vi "GetFrame.vi"(8 "error in (no error)":errorcluster, 11 "ZWO_ASI in":refnum<class "ZWO_ASI.lvclass">) -> (0 "error out":errorcluster, 3 "ZWO_ASI out":refnum<class "ZWO_ASI.lvclass">)   [LabVIEW 2023, in "ZWO_ASI.lvlib" / "ZWO_ASI.lvclass"]
uses:
  ZWO_ASI.lvclass
  Labview_ASI_demo_64bit_221128/user.lib/ASICamera2_no_err/ASICamera2_no_err.lvlib
  <vilib>/ActorFramework/Actor/Actor.lvclass
  ZWO_ASI Messages/GetFrame Msg/GetFrame Msg.lvclass
  C:/Program Files/National Instruments/LabVIEW 2023/vi.lib/ActorFramework/Actor/Actor.lvclass
  C:/Users/quantum/Documents/LVDAQ/ConcreteClasses/ConcreteInstrumentClasses/CameraClasses/ZWO_ASI_LV/ZWO_ASI/ZWO_ASI.lvclass
  C:/Users/quantum/Documents/LVDAQ/Interfaces/AbstractInstrumentClasses/Cameras_LV/CameraInterface/CameraInterface.lvclass
  C:/Users/quantum/Documents/LVDAQ/Interfaces/InitDeinitInterface/InitDeinit/InitDeinit.lvclass
  ZWO_ASI Messages/StopCapture Msg/StopCapture Msg.lvclass
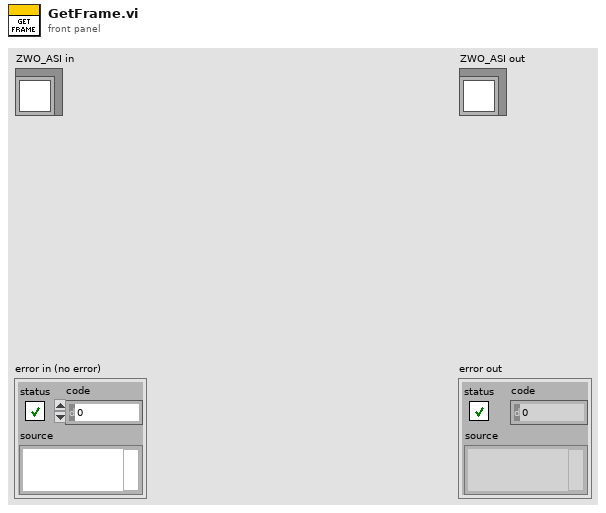
[diagram p1: front panel]
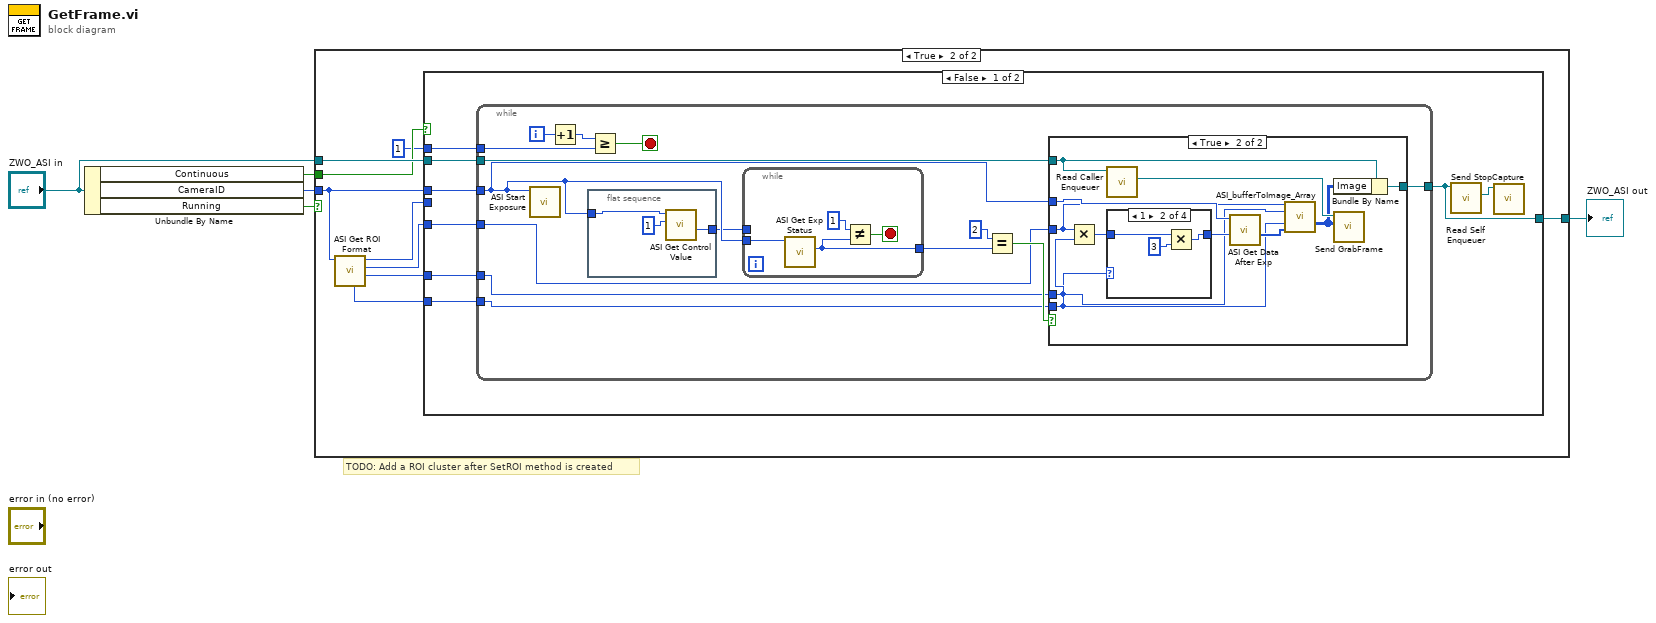
[diagram p0: block diagram]
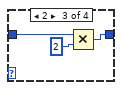
[diagram p5: hidden frame]
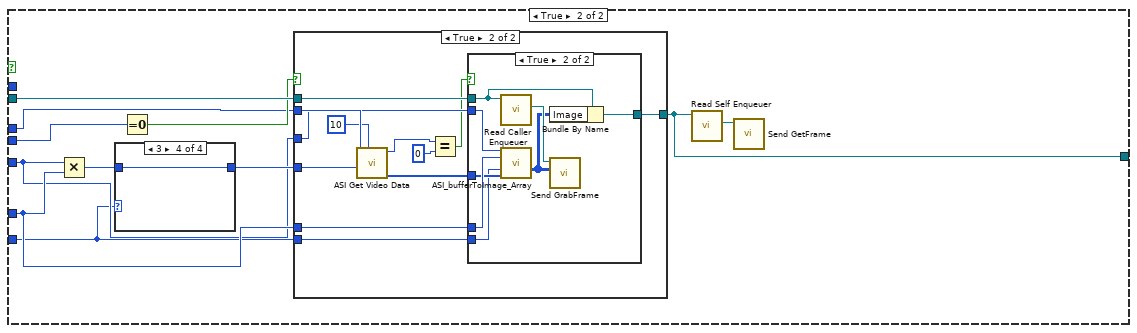
[diagram p7: hidden frame]
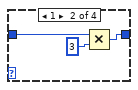
[diagram p11: hidden frame]
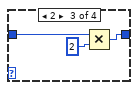
[diagram p12: hidden frame]
diagram:
  # "TODO: Add a ROI cluster after SetROI method is created"
  n1 = Unbundle By Name("ZWO_ASI in") -> ("Continuous"=w4:bool, "CameraID"=w3:i32, "Running"=w2:bool)
  n2 = case shown="True" w2 {
    tunnel: "ZWO_ASI in" -> [w6 w15]
    tunnel: [w6 w14] -> w1
    tunnel: w4 -> [_ w9]
    tunnel: w3 -> [_ w8]
    frame False {
    }
    frame True {
      n3 = call "ASI Get ROI Format.vi"("iCameraID"=w8) -> ("piHeight out"=w13:i32, "piWidth out"=w10:i32, "function return"=w12:i32, "pImg_type out"=w11:i32)  [unwired: 6 in, 1 out]
      n4 = case shown="False" w9 {
        tunnel: w15 -> [w19 w75]
        tunnel: [w17 w65] -> w14
        tunnel: w13 -> [w21 w71]
        tunnel: w10 -> [w20 w70]
        tunnel: w12 -> [_ w69]
        tunnel: w11 -> [w22 w68]
        tunnel: w8 -> [w23 w67]
        tunnel: 1 ("num of frames") -> [w18 _]
        frame False {
          n5 = while {
            tunnel: w23 -> [w36]
            tunnel: w20 -> [w33]
            tunnel: w22 -> [w28]
            tunnel: w21 -> [w29]
            tunnel: w19 -> [w27]
            tunnel: [w26] -> w17
            tunnel: w18 -> [w25]
            i -> [w35]
            stop <- w24 stop-if-true
            n6 = call "ASI Start Exposure.vi"("iCameraID"=w36) -> ()  [unwired: 10 in, 1 out]
            n7 = Increment(x=w35) -> (x+1=w34:i32)
            n8 = flat-sequence {
              tunnel: w36 -> [w40]
              tunnel: [w39] -> w32
              frame #0 {
                n9 = call "ASI Get Control Value.vi"("ControlType"=1, "iCameraID"=w40) -> ("plValue out"=w39:i32)  [unwired: 7 in, 2 out]
              }
            }
            n10 = Greater Or Equal?(x=w34, y=w25) -> (x >= y?=w24:bool)
            n11 = while {
              tunnel: w36 -> [w44]
              tunnel: [w41] -> w31
              tunnel: w32 -> [_]
              stop <- w42 stop-if-true
              n12 = call "ASI Get Exp Status.vi"("iCameraID"=w44) -> ("pExpStatus out"=w41:u32)  [unwired: 9 in, 1 out]
              n13 = Not Equal?(x=u32 1, y=w41) -> (x != y?=w42:bool)
            }
            n14 = Equal?(x=u32 2, y=w31) -> (x = y?=w37:bool)
            n15 = case shown="True" w37 {
              tunnel: w36 -> [_ w56]
              tunnel: w33 -> [_ w51]
              tunnel: w29 -> [_ w52]
              tunnel: w28 -> [_ w50]
              tunnel: w27 -> [w45 w46]
              tunnel: [w45 w49] -> w26
              frame False {
              }
              frame True {
                n16 = Multiply(x=w51, y=w52) -> (x*y=w54:i32)
                n17 = call <vilib>:"Read Caller Enqueuer.vi"("Actor"=w46) -> ("Caller Enqueuer"=w48:refnum<class "Message Enqueuer.lvclass">)  [unwired: 10 in]
                n18 = case shown="1" w50 {
                  tunnel: w54 -> [w57 w60 w63 w64]
                  tunnel: [w57 w58 w61 w64] -> w55
                  frame 0, Default {
                  }
                  frame 1 {
                    n19 = Multiply(x=w60, y=3) -> (x*y=w58:i32)
                  }
                  frame 2 {
                    n20 = Multiply(x=w63, y=2) -> (x*y=w61:i32)
                  }
                  frame 3 {
                  }
                }
                n21 = call "ASI Get Data After Exp.vi"("lBuffSize"=w55, "iCameraID"=w56) -> ("pBuffer out"=w53:u8[])  [unwired: 8 in, 1 out]
                n22 = call "ASI_bufferToImage_Array.vi"("iWidth"=w51, "iHeight"=w52, "imageType"=w50, "pBuffer in"=w53) -> ("output array"=w47:u32[][])  [unwired: 11 in]
                n23 = Bundle By Name(cluster=w46, "Image"=w47) -> (w49:refnum<class "ZWO_ASI.lvclass">)
                n24 = call "Send GrabFrame.vi"("Image"=w47, "Message Enqueuer"=w48) -> ()  [unwired: 8 in, 2 out]
              }
            }
          }
          n25 = call <vilib>:"Read Self Enqueuer.vi"("Actor"=w17) -> ("Self Enqueuer"=w16:refnum<class "Message Enqueuer.lvclass">)  [unwired: 10 in]
          n26 = call "Send StopCapture.vi"("Message Enqueuer"=w16) -> ()  [unwired: 9 in, 2 out]
        }
        frame True {
          n27 = Multiply(x=w70, y=w71) -> (x*y=w73:i32)
          n28 = case shown="3" w68 {
            tunnel: w73 -> [w98 w101 w104 w105]
            tunnel: [w98 w99 w102 w105] -> w74
            frame 0, Default {
            }
            frame 1 {
              n29 = Multiply(x=w101, y=3) -> (x*y=w99:i32)
            }
            frame 2 {
              n30 = Multiply(x=w104, y=2) -> (x*y=w102:i32)
            }
            frame 3 {
            }
          }
          n31 = Equal To 0?(x=w69) -> (x = 0?=w72:bool)
          n32 = case shown="True" w72 {
            tunnel: w67 -> [_ w88]
            tunnel: w75 -> [w76 w87]
            tunnel: [w76 w86] -> w65
            tunnel: w68 -> [_ w85]
            tunnel: w71 -> [_ w84]
            tunnel: w70 -> [_ w83]
            tunnel: w74 -> [_ w82]
            frame False {
            }
            frame True {
              n33 = call "ASI Get Video Data.vi"("iWaitms"=10, "lBuffSize"=w82, "iCameraID"=w88) -> ("pBuffer out"=w80:u8[], "function return"=w79:i32)  [unwired: 7 in]
              n34 = Equal?(x=w79, y=0) -> (x = y?=w77:bool)
              n35 = case shown="True" w77 {
                tunnel: w83 -> [_ w97]
                tunnel: w84 -> [_ w96]
                tunnel: w80 -> [_ w95]
                tunnel: w85 -> [_ w94]
                tunnel: w87 -> [w89 w90]
                tunnel: [w89 w93] -> w86
                frame False {
                }
                frame True {
                  n36 = call <vilib>:"Read Caller Enqueuer.vi"("Actor"=w90) -> ("Caller Enqueuer"=w92:refnum<class "Message Enqueuer.lvclass">)  [unwired: 10 in]
                  n37 = call "ASI_bufferToImage_Array.vi"("iWidth"=w97, "iHeight"=w96, "imageType"=w94, "pBuffer in"=w95) -> ("output array"=w91:u32[][])  [unwired: 11 in]
                  n38 = Bundle By Name(cluster=w90, "Image"=w91) -> (w93:refnum<class "ZWO_ASI.lvclass">)
                  n39 = call "Send GrabFrame.vi"("Image"=w91, "Message Enqueuer"=w92) -> ()  [unwired: 8 in, 2 out]
                }
              }
            }
          }
          n40 = call <vilib>:"Read Self Enqueuer.vi"("Actor"=w65) -> ("Self Enqueuer"=w66:refnum<class "Message Enqueuer.lvclass">)  [unwired: 10 in]
          n41 = call "Send GetFrame.vi"("Message Enqueuer"=w66) -> ()  [unwired: 9 in, 2 out]
        }
      }
    }
  }
  "ZWO_ASI out" <- w1
